vi "SRV_Format and Write Diagnostic Log.vi"(7 "error to log":errorcluster, 11 "error in (no error)":errorcluster) -> (15 "error out":errorcluster)   [LabVIEW 2014]
uses:
  <vilib>/Utility/sysdir.llb/System Directory Type.ctl
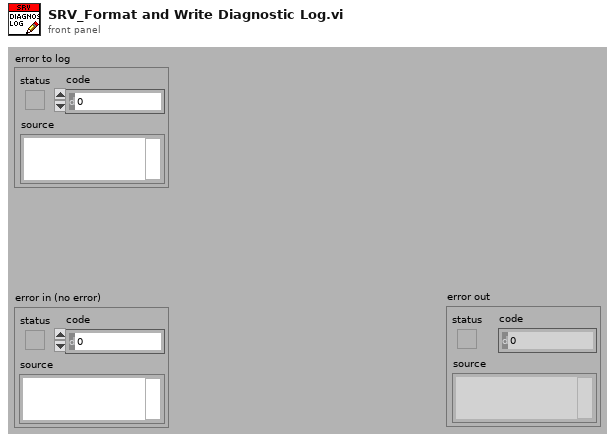
[diagram p1: front panel]
types:
  T1 = typedef "System Directory Type.ctl" = i32
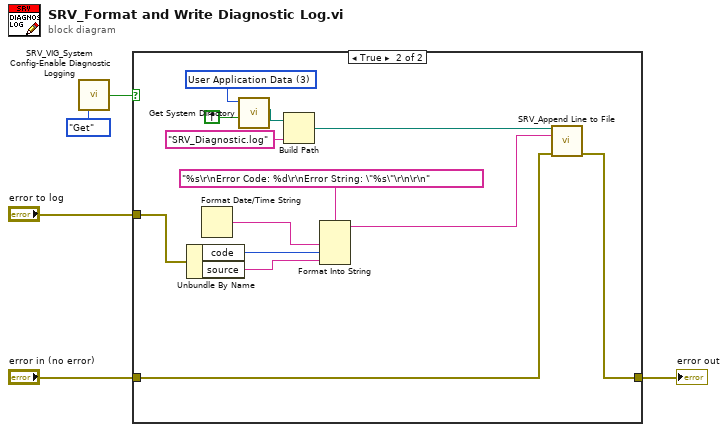
[diagram p0: block diagram]
diagram:
  n1 = call "SRV_VIG_System Config-Enable Diagnostic Logging.vi"("Method (Get)"=enum16{"Get", "Set"}."Get") -> ("Enable Diagnostic Log?"=w4:bool)  [unwired: 14 in]
  n2 = case shown="True" w4 {
    tunnel: "error to log" -> [_ w13]
    tunnel: "error in (no error)" -> [w6 w14]
    tunnel: [w6 w8] -> w2
    frame False {
    }
    frame True {
      w19 = T1 3 items=["User Home", "User Desktop", "User Documents", "User Application Data", "User Preferences", "User Temporary", "Public Documents", "Public Application Data", "Public Preferences", "System Core Libraries", "System Installed Libraries", "Application Files", "Boot Volume Root"] ("system directory type")
      n3 = Unbundle By Name(w13) -> ("code"=w11:i32, "source"=w10:string)
      n4 = Format Date/Time String() -> (date/time string=w9:string)  [unwired: 3 in]
      n5 = call <vilib>:"Get System Directory.vi"("create directory if not found? (F)"=TRUE, "system directory type"=w19) -> ("system directory"=w18:path)  [unwired: 9 in]
      n6 = Build Path(base path=w18, name or relative path="SRV_Diagnostic.log") -> (appended path=w15:path)
      n7 = Format Into String(format string="%s\r\nError Code: %d\r\nError String: \"%s\"\r\n\r\n", w9, w11, w10) -> (resulting string=w7:string)  [unwired: 2 in, 1 out]
      n8 = call "SRV_Append Line to File.vi"("file path"=w15, "Line to Write"=w7, "error in (no error)"=w14) -> ("error out"=w8:errorcluster)  [unwired: 12 in]
    }
  }
  "error out" <- w2
